vi "_OBSOLETE_PathPlanner_Trajectory_CalculateMaxVel.vi"(8 "Reversed":bool, 9 "MaxAccel":dbl, 10 "MaxVel":dbl, 11 "PathPlannerStates":T1[](array[typedef]) {"TargetHolonomicRotation"."SIN" format="%13.4f"; "TargetHolonomicRotation"."COS" format="%13.4f"; "TargetHolonomicRotation"."VALUE" format="%13.4f"; "Heading"."SIN" format="%13.4f"; "Heading"."COS" format="%13.4f"; "Heading"."VALUE" format="%13.4f"; "PositionMeters"."Y" format="%14.3f"; "PositionMeters"."X" format="%14.3f"}) -> (3 "outPathPlannerStates":T1[](array[typedef]) {"TargetHolonomicRotation"."SIN" format="%13.4f"; "TargetHolonomicRotation"."COS" format="%13.4f"; "TargetHolonomicRotation"."VALUE" format="%13.4f"; "Heading"."SIN" format="%13.4f"; "Heading"."COS" format="%13.4f"; "Heading"."VALUE" format="%13.4f"; "PositionMeters"."Y" format="%14.3f"; "PositionMeters"."X" format="%14.3f"})   [LabVIEW 2019]
uses:
  <vilib>/Rock Robotics/WPI/ThirdParty/JAS_Junk/TrajLib/TypeDef/ROTATION2D.ctl
  <vilib>/Rock Robotics/WPI/ThirdParty/JAS_Junk/TrajLib/Trajectory_Library.lvlib
  <vilib>/Rock Robotics/WPI/ThirdParty/JAS_Junk/TrajLib/TypeDef/TRANSLATION2D.ctl
  TypeDef/PathPlannerTrajectoryState.ctl
  PathPlanner24.lvlib
  TypeDef/PathPlannerPathConstraints.ctl
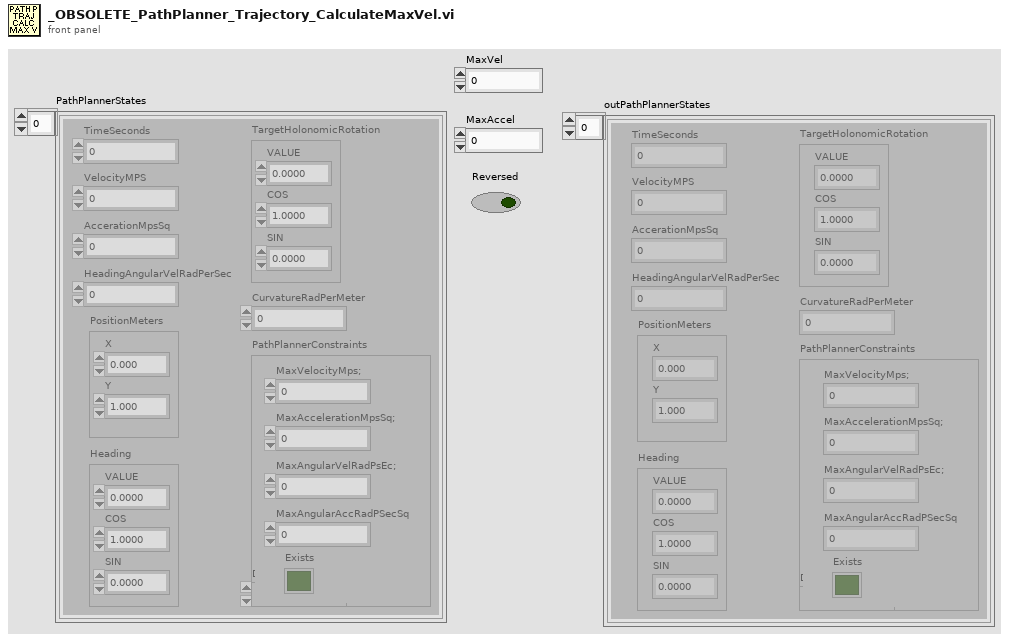
[diagram p1: front panel]
types:
  T1 = typedef "PathPlanner24.lvlib/PathPlannerTrajectoryState.ctl" = cluster{"TimeSeconds":dbl, "VelocityMPS":dbl, "AccerationMpsSq":dbl, "HeadingAngularVelRadPerSec":dbl, "PositionMeters":T2, "Heading":T3, "TargetHolonomicRotation":T3, "CurvatureRadPerMeter":dbl, "DeltaPos":dbl, "PathPlannerConstraints":T4}
  T2 = typedef "Trajectory_Library.lvlib/TRANSLATION2D.ctl" = cluster{"X":dbl, "Y":dbl}
  T3 = typedef "Trajectory_Library.lvlib/ROTATION2D.ctl" = cluster{"VALUE":dbl, "COS":dbl, "SIN":dbl}
  T4 = typedef "PathPlanner24.lvlib/PathPlannerPathConstraints.ctl" = cluster{"MaxVelocityMps;":dbl, "MaxAccelerationMpsSq;":dbl, "MaxAngularVelRadPsEc;":dbl, "MaxAngularAccRadPSecSq":dbl, "Exists":bool}
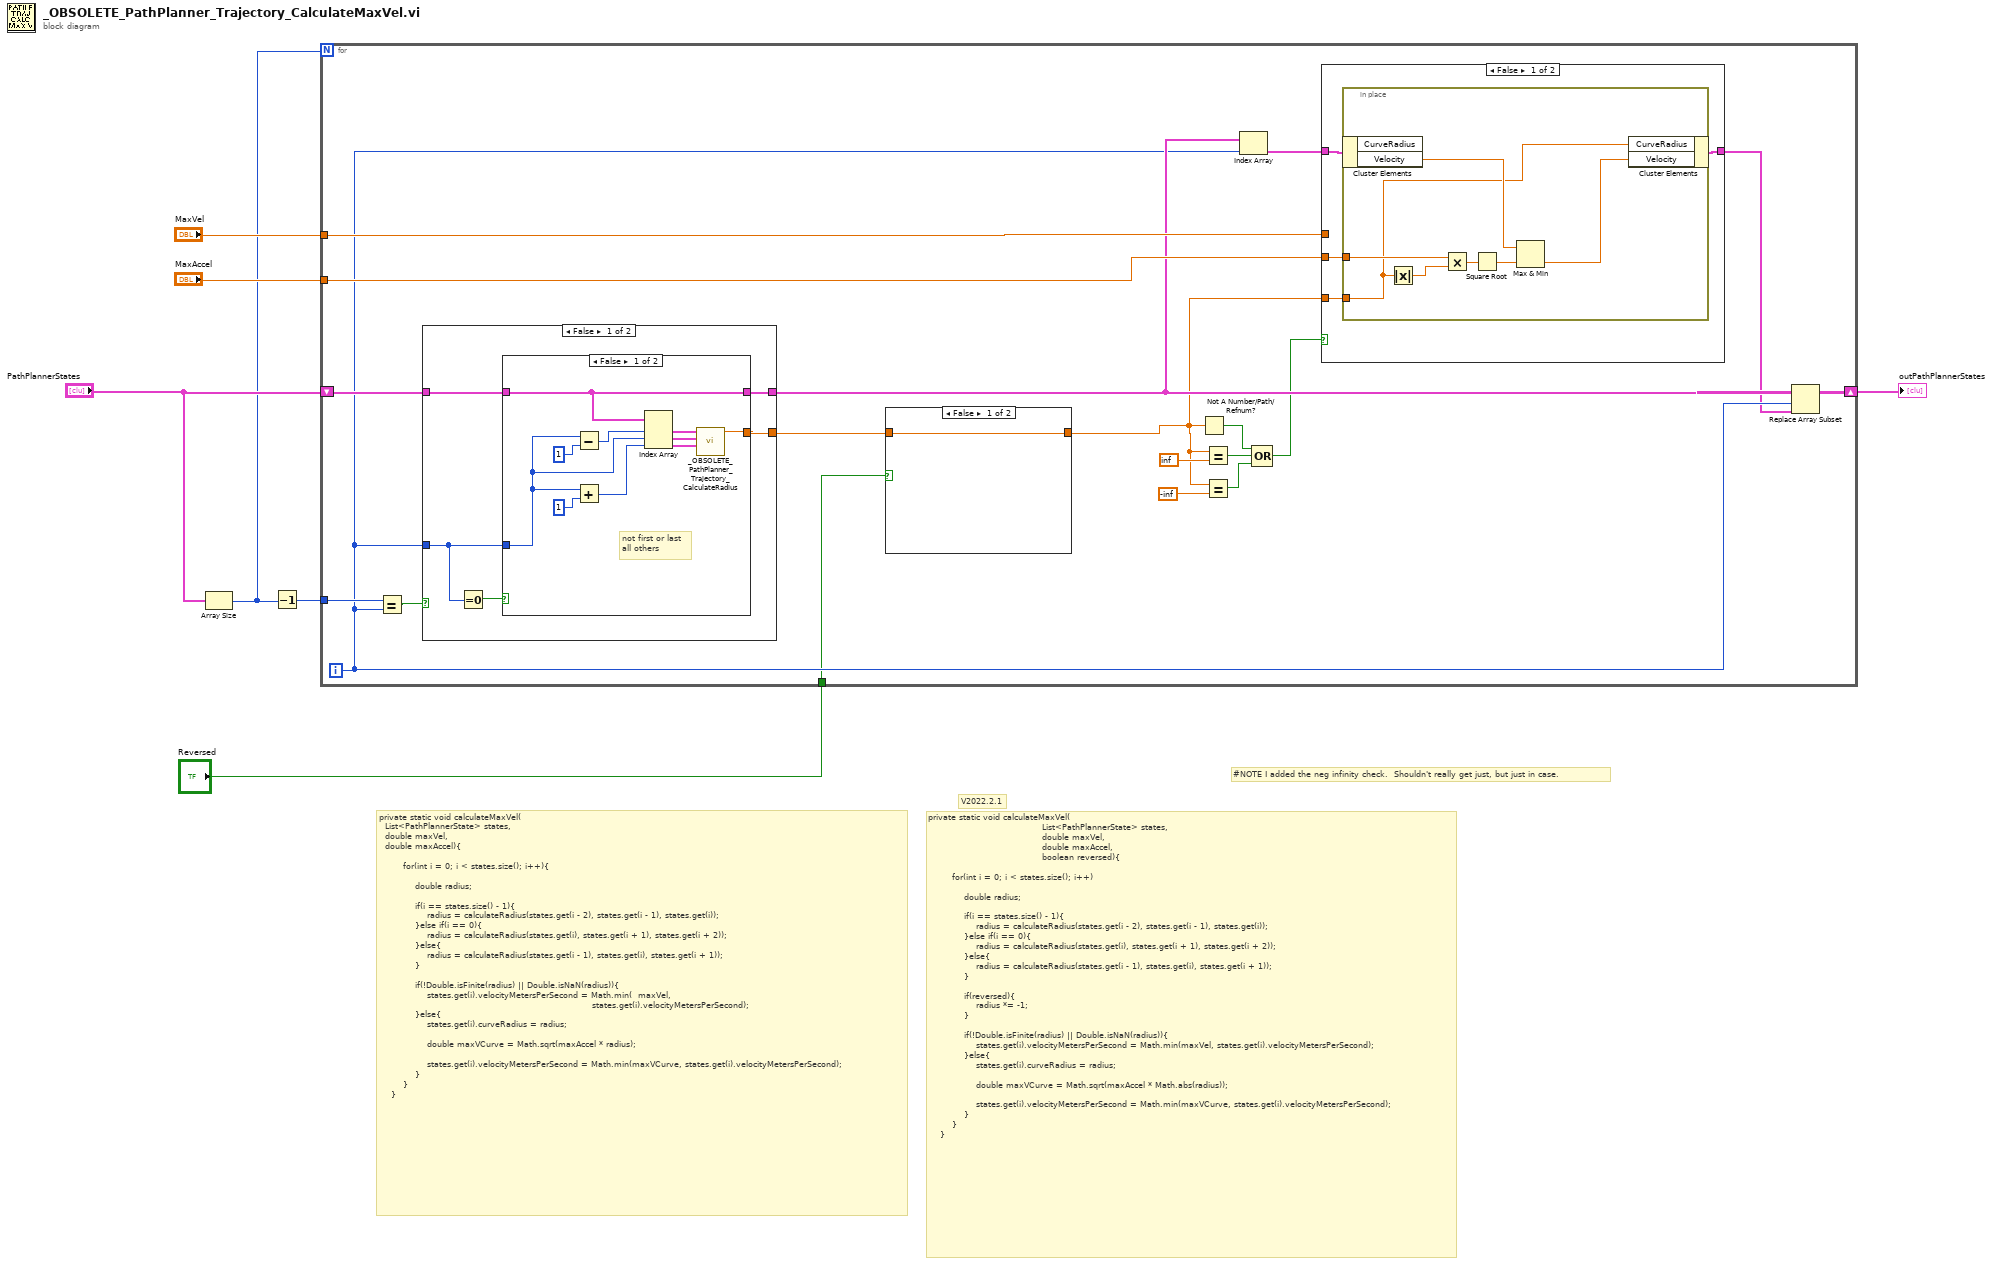
[diagram p0: block diagram]
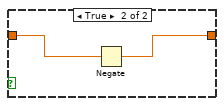
[diagram p2: hidden frame]
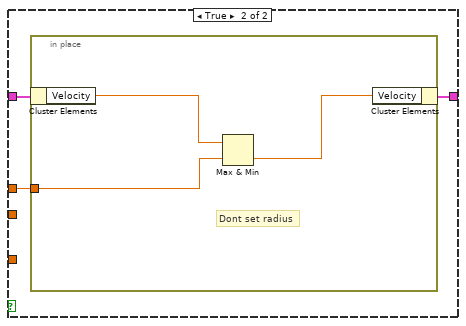
[diagram p3: hidden frame]
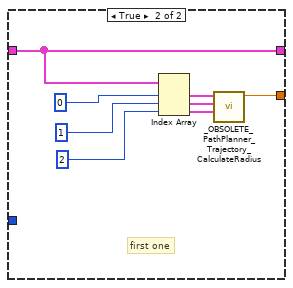
[diagram p4: hidden frame]
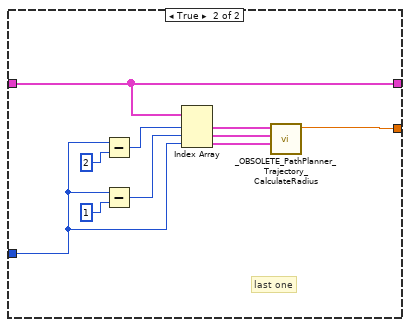
[diagram p5: hidden frame]
diagram:
  # "V2022.2.1"
  # "private static void calculateMaxVel(\n                                      List<PathPlannerState> states, \n                                      double maxVel, \n                                      double maxAccel, \n                                      boolean reversed){\n\n        for(int i = 0; i < states.size(); i++)\n\n            double radius;\n\n            if(i == states.size() - 1){\n                radius = calculateRadius(states.get(i - 2), states.get(i - 1), states.get(i));\n            }else if(i == 0){\n                radius = calculateRadius(states.get(i), states.get(i + 1), states.get(i + 2));\n            }else{\n                radius = calculateRadius(states.get(i - 1), states.get(i), states.get(i + 1));\n            }\n\n            if(reversed){\n                radius *= -1;\n            }\n\n            if(!Double.isFinite(radius) || Double.isNaN(radius)){\n                states.get(i).velocityMetersPerSecond = Math.min(maxVel, states.get(i).velocityMetersPerSecond);\n            }else{\n                states.get(i).curveRadius = radius;\n\n                double maxVCurve = Math.sqrt(maxAccel * Math.abs(radius));\n\n                states.get(i).velocityMetersPerSecond = Math.min(maxVCurve, states.get(i).velocityMetersPerSecond);\n            }\n        }\n    }"
  # "private static void calculateMaxVel(\n\t\tList<PathPlannerState> states, \n\t\tdouble maxVel, \n\t\tdouble maxAccel){\n\n        for(int i = 0; i < states.size(); i++){\n\n            double radius;\n\n            if(i == states.size() - 1){\n                radius = calculateRadius(states.get(i - 2), states.get(i - 1), states.get(i));\n            }else if(i == 0){\n                radius = calculateRadius(states.get(i), states.get(i + 1), states.get(i + 2));\n            }else{\n                radius = calculateRadius(states.get(i - 1), states.get(i), states.get(i + 1));\n            }\n\n            if(!Double.isFinite(radius) || Double.isNaN(radius)){\n                states.get(i).velocityMetersPerSecond = Math.min(  maxVel, \n\t\t\t\t                                                                   states.get(i).velocityMetersPerSecond);\n            }else{\n                states.get(i).curveRadius = radius;\n\n                double maxVCurve = Math.sqrt(maxAccel * radius);\n\n                states.get(i).velocityMetersPerSecond = Math.min(maxVCurve, states.get(i).velocityMetersPerSecond);\n            }\n        }\n    }"
  # "#NOTE I added the neg infinity check.  Shouldn't really get just, but just in case."
  n1 = Array Size(array="PathPlannerStates") -> (size(s)=w2:i32)
  n2 = Decrement(x=w2) -> (x-1=w7:i32)
  n3 = for {
    N: w2 -> [_]
    tunnel: w7 -> [w26]
    tunnel: "MaxVel" -> [w18]
    tunnel: "MaxAccel" -> [w17]
    shift-right: [w15] -> w3
    shift-left: "PathPlannerStates" -> [w24]
    tunnel: "Reversed" -> [w8]
    i -> [w13]
    n4 = Equal?(x=w26, y=w13) -> (x = y?=w25:bool)
    n5 = case shown="False" w25 {
      tunnel: w24 -> [w50 w70]
      tunnel: w13 -> [w48 w75]
      tunnel: [w49 w71] -> w10
      tunnel: [w47 w70] -> w14
      frame False {
        n6 = Equal To 0?(x=w48) -> (x = 0?=w51:bool)
        n7 = case shown="False" w51 {
          tunnel: w50 -> [w52 w62]
          tunnel: [w53 w63] -> w49
          tunnel: w48 -> [w55 _]
          tunnel: [w52 w62] -> w47
          frame False {
            # "not first or last\nall others"
            n8 = Subtract(x=w55, y=1) -> (x-y=w59:i32)
            n9 = Add(x=w55, y=1) -> (x+y=w54:i32)
            n10 = Index Array(array=w52, index #1=w59, index #2=w55, index #3=w54) -> (element #1=w58:T1, element #2=w57:T1, element #3=w56:T1)
            n11 = call "_OBSOLETE_PathPlanner_Trajectory_CalculateRadius.vi"("S2"=w56, "S1"=w57, "S0"=w58) -> ("Radius"=w53:dbl)  [unwired: 8 in]
          }
          frame True {
            # "first one"
            n12 = Index Array(array=w62, index #1=0 ("y"), index #2=1 ("y"), index #3=2 ("y")) -> (element #1=w69:T1, element #2=w68:T1, element #3=w67:T1)
            n13 = call "_OBSOLETE_PathPlanner_Trajectory_CalculateRadius.vi"("S2"=w67, "S1"=w68, "S0"=w69) -> ("Radius"=w63:dbl)  [unwired: 8 in]
          }
        }
      }
      frame True {
        # "last one"
        n14 = Subtract(x=w75, y=2) -> (x-y=w77:i32)
        n15 = Subtract(x=w75, y=1) -> (x-y=w76:i32)
        n16 = Index Array(array=w70, index #1=w77, index #2=w76, index #3=w75) -> (element #1=w74:T1, element #2=w73:T1, element #3=w72:T1)
        n17 = call "_OBSOLETE_PathPlanner_Trajectory_CalculateRadius.vi"("S2"=w72, "S1"=w73, "S0"=w74) -> ("Radius"=w71:dbl)  [unwired: 8 in]
      }
    }
    n18 = case shown="False" w8 {
      tunnel: w10 -> [w27 w29]
      tunnel: [w27 w28] -> w9
      frame False {
      }
      frame True {
        n19 = Negate(x=w29) -> (-x=w28:dbl)
      }
    }
    n20 = Not A Number/Path/Refnum?(number/path/refnum=w9) -> (NaN/Path/Refnum?=w21:bool)
    n21 = Equal?(x=w9, y=inf) -> (x = y?=w20:bool)
    n22 = Equal?(x=w9, y=-inf) -> (x = y?=w19:bool)
    n23 = Index Array(array=w14, index=w13) -> (element=w16:T1)
    n24 = Compound Arithmetic op=OR(w21, w20, w19) -> (w11:bool)
    n25 = case shown="False" w11 {
      tunnel: [w33 w43] -> w12
      tunnel: w18 -> [_ w42]
      tunnel: w9 -> [w32 _]
      tunnel: w17 -> [w31 _]
      tunnel: w16 -> [w30 w41]
      frame False {
        n26 = in-place {
          in-place-border: w32 -> [w35]
          in-place-border: w31 -> [w40]
          n27 = in-place-cluster #1(w30) -> ("Velocity"=w36:dbl)  [unwired: 1 out]
          n28 = Absolute Value(x=w35) -> (abs(x)=w34:dbl)
          n29 = Multiply(x=w40, y=w34) -> (x*y=w39:dbl)
          n30 = Square Root(x=w39) -> (sqrt(x)=w38:dbl)
          n31 = Max & Min(x=w36, y=w38) -> (min(x,y)=w37:dbl)  [unwired: 1 out]
          n32 = in-place-cluster #1("CurveRadius"=w35, "Velocity"=w37) -> (w33:T1)
        }
      }
      frame True {
        n33 = in-place {
          in-place-border: w42 -> [w45]
          # "Dont set radius"
          n34 = in-place-cluster #2(w41) -> ("Velocity"=w44:dbl)
          n35 = Max & Min(x=w44, y=w45) -> (min(x,y)=w46:dbl)  [unwired: 1 out]
          n36 = in-place-cluster #2("Velocity"=w46) -> (w43:T1)
        }
      }
    }
    n37 = Replace Array Subset(array=w14, new element=w12, index=w13) -> (w15:T1[])
  }
  "outPathPlannerStates" <- w3
